vi "Spectrum Analyzer.vi"() -> ()   [LabVIEW 2024]
uses:
  <vilib>/express/express analysis/Spectral/Block/exnSpectralBlock spectral measurements RMS poly.vi
  <vilib>/express/express analysis/Spectral/Block/exnSpectralBlock spectral measurements power poly.vi
  <vilib>/express/express analysis/Spectral/XNode/ExpressSpectralMeasurementsBlockNode.xnode
  <vilib>/express/express analysis/Spectral/Block/exnSpectralBlock spectral measurements power DDT.vi
  <vilib>/express/express analysis/Spectral/Block/exnSpectralBlock spectral measurements RMS DDT.vi
panel:
  out "Raw Data":dynamicdata(graph)
  out "FFT":dynamicdata(graph)
  out "Power Spectrum":dynamicdata(graph)
  in  "Simulated Inputs":T1(ring)
  # "Choose what input you want from drop down menu"
  # "Power Spectrum"
  # "FFT"
  # "Raw Data"
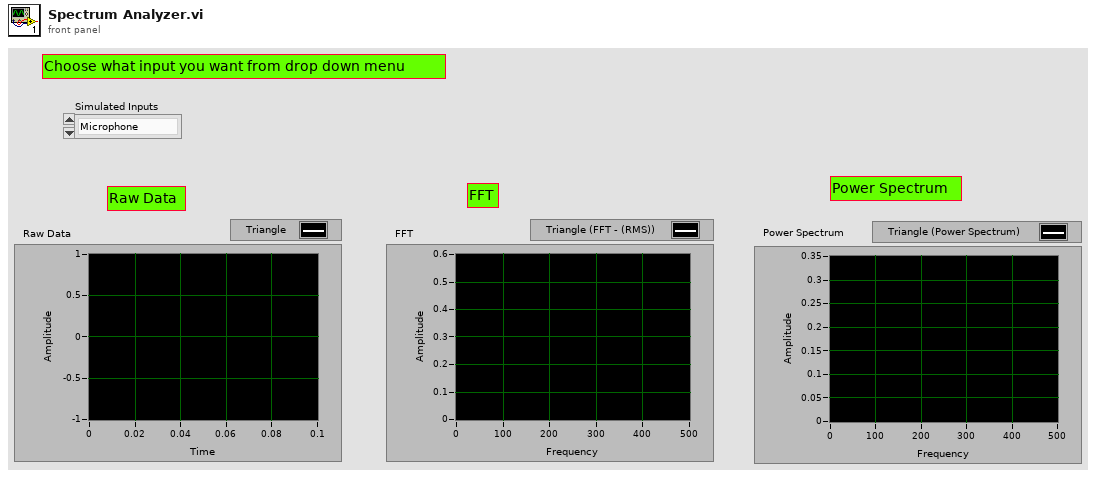
[diagram p1: front panel]
types:
  T1 = enum16{"Microphone", "Sin", "Cos", "Square", "Triangle"}
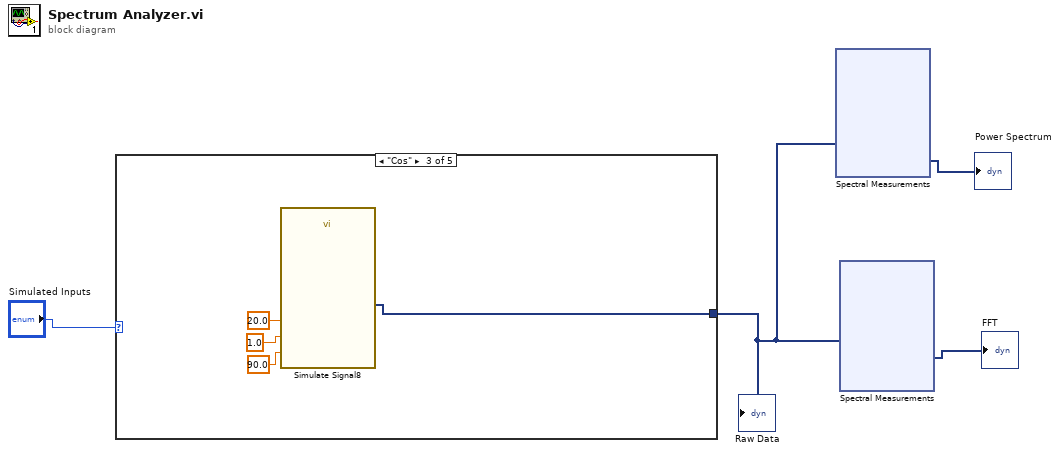
[diagram p0: block diagram]
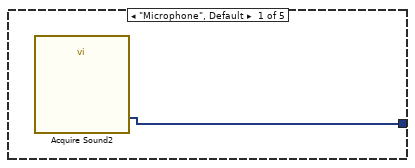
[diagram p2: hidden frame]
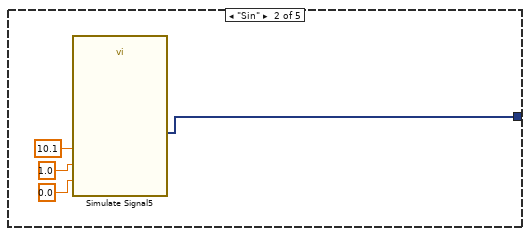
[diagram p3: hidden frame]
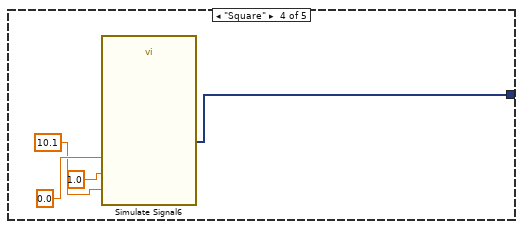
[diagram p4: hidden frame]
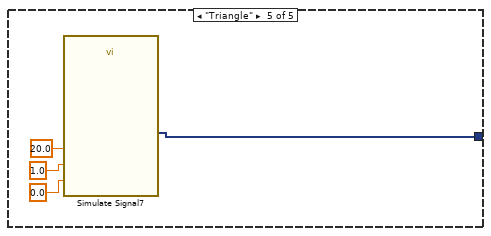
[diagram p5: hidden frame]
diagram:
  n1 = case shown="\"Cos\"" "Simulated Inputs" {
    tunnel: [w5 w9 w11 w17 w21] -> w2
    frame "Microphone", Default {
      n2 = call "Acquire Sound2"() -> ("Data"=w5:dynamicdata)  [unwired: 18 in, 1 out]
    }
    frame "Sin" {
      n3 = call "Simulate Signal5"("Frequency"=10.1, "Amplitude"=1.0, "Phase"=0.0) -> ("Sine"=w9:dynamicdata)  [unwired: 11 in, 1 out]
    }
    frame "Cos" {
      n4 = call "Simulate Signal8"("Frequency"=20.0, "Amplitude"=1.0, "Phase"=90.0) -> ("Sine"=w11:dynamicdata)  [unwired: 11 in, 1 out]
    }
    frame "Square" {
      n5 = call "Simulate Signal6"("Frequency"=10.1, "Amplitude"=1.0, "Phase"=0.0) -> ("Square"=w17:dynamicdata)  [unwired: 11 in, 1 out]
    }
    frame "Triangle" {
      n6 = call "Simulate Signal7"("Frequency"=20.0, "Amplitude"=1.0, "Phase"=0.0) -> ("Triangle"=w21:dynamicdata)  [unwired: 11 in, 1 out]
    }
  }
  "Raw Data" <- w2
  n7 = xnode "Spectral Measurements"("Signals"=w2) -> ("Power Spectrum"=→"Power Spectrum":dynamicdata)  [unwired: 1 in, 1 out]
  n8 = xnode "Spectral Measurements"("Signals"=w2) -> ("FFT - (RMS)"=→"FFT":dynamicdata)  [unwired: 1 in, 2 out]
